vi "Not Opening Tag.vi"(8 "Error In":errorcluster, 11 "Parser In":refnum<class "Parser.lvclass">) -> (0 "Error Out":errorcluster, 3 "Parser Out":refnum<class "Parser.lvclass">)   [LabVIEW 2017, in "Mustache.lvlib" / "Parser.lvclass"]
uses:
  Parser.lvclass
  Parser.lvclass/Parser.ctl
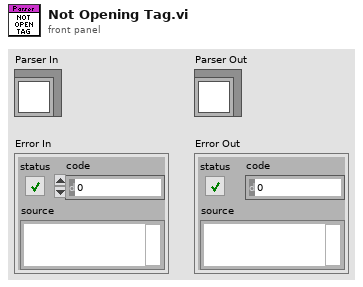
[diagram p1: front panel]
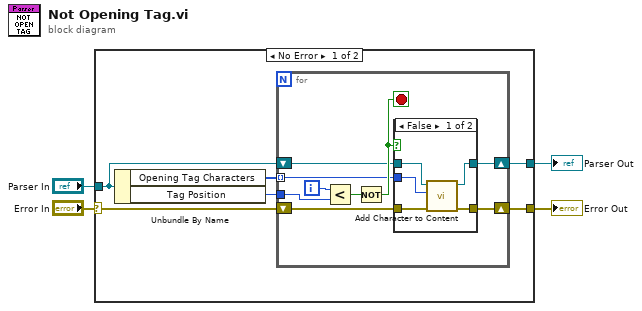
[diagram p0: block diagram]
diagram:
  n1 = case shown="No Error" "Error In" {
    selector: "Error In" -> [w9 w28]
    tunnel: [w5 w28] -> w3
    tunnel: "Parser In" -> [w7 w27]
    tunnel: [w6 w27] -> w1
    frame No Error {
      n2 = Unbundle By Name(w7) -> ("Opening Tag Characters"=w10:u8[], "Tag Position"=w8:i32)
      n3 = for {
        tunnel: w10 -> [w11] mode=indexing
        tunnel: w8 -> [w18]
        shift-right: [w14] -> w6
        shift-left: w7 -> [w15]
        shift-right: [w12] -> w5
        shift-left: w9 -> [w13]
        i -> [w19]
        stop <- w16 stop-if-true
        n4 = Less?(x=w19, y=w18) -> (x < y?=w17:bool)
        n5 = Not(x=w17) -> (.not. x?=w16:bool)
        n6 = case shown="False" w16 {
          tunnel: w15 -> [w24 w26]
          tunnel: [w23 w26] -> w14
          tunnel: w13 -> [w22 w25]
          tunnel: [w21 w25] -> w12
          tunnel: w11 -> [w20 _]
          frame False {
            n7 = call "Add Character to Content.vi"("Error In"=w22, "Character"=w20, "Parser In"=w24) -> ("Error Out"=w21:errorcluster, "Parser Out"=w23:refnum<class "Parser.lvclass">)  [unwired: 7 in]
          }
          frame True {
          }
        }
      }
    }
    frame Error {
    }
  }
  "Error Out" <- w3
  "Parser Out" <- w1
